vi "set IR test parameters.vi"(7 "IR Parameters":T1={"Voltage Level [V]"=1000, "Hi Limit [ohm]"=2500000.0, "Test Time [s] "=3.3, "Dwell Time [s]"=4.4, "Lo Limit [ohm]"=30000000000.0, "Ramp Time [s] "=1.1, "Fall Time [s]"=2.2} {"Voltage Level [V]" format="%.3p"; "Hi Limit [ohm]" format="%#_6p"; "Lo Limit [ohm]" format="%#_6p"}, 8 "error in (no error)":errorcluster, 10 "Step":T2 min=1 max=99 step=1, 11 "VISA Refnum in":refnum<visa-resource-name>) -> (0 "error out":errorcluster, 3 "VISA Refnum out":refnum<visa-resource-name>)   [LabVIEW 2025]
uses:
  Type Def/steps--ring.ctl
  Type Def/AC-DC-IR modes--ring.ctl
  Type Def/DC-IR modes--ring.ctl
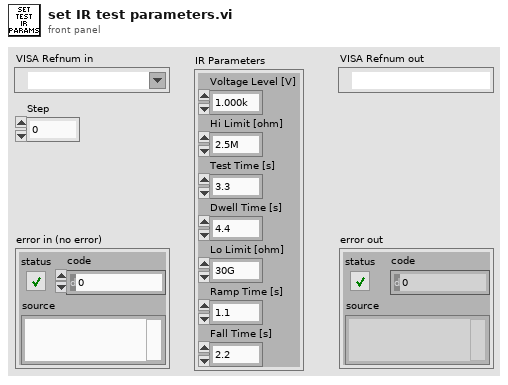
[diagram p1: front panel]
types:
  T1 = cluster{"Voltage Level [V]":u16, "Hi Limit [ohm]":dbl, "Test Time [s] ":dbl, "Dwell Time [s]":dbl, "Lo Limit [ohm]":dbl, "Ramp Time [s] ":dbl, "Fall Time [s]":dbl}
  T2 = typedef "steps--ring.ctl" = u8
  T3 = typedef "DC-IR modes--ring.ctl" = u16
  T4 = typedef "AC-DC-IR modes--ring.ctl" = u16
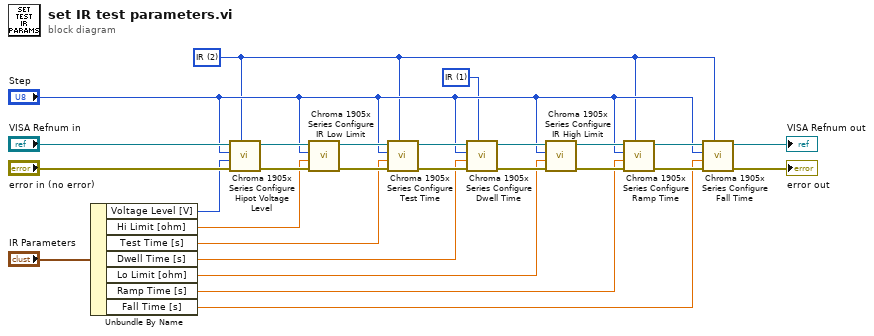
[diagram p0: block diagram]
diagram:
  w10 = T3 1 items=["DC", "IR"] ("Mode")
  w9 = T4 2 items=["AC", "DC", "IR"] ("Mode")
  n1 = Unbundle By Name("IR Parameters") -> ("Voltage Level [V]"=w7:u16, "Hi Limit [ohm]"=w6:dbl, "Test Time [s]"=w5:dbl, "Dwell Time [s]"=w4:dbl, "Lo Limit [ohm]"=w3:dbl, "Ramp Time [s]"=w2:dbl, "Fall Time [s]"=w1:dbl)
  n2 = call "Chroma 1905x Series Configure Hipot Voltage Level.vi"("Mode"=w9, "error in (no error)"="error in (no error)", "Voltage Level [V]"=w7, "Step"="Step", "VISA resource name"="VISA Refnum in") -> ("error out"=w18:errorcluster, "VISA resource name out"=w15:refnum<visa-resource-name>)  [unwired: 5 in]
  n3 = call "Chroma 1905x Series Configure IR Low Limit.vi"("error in (no error)"=w18, "Low Limit [ohm]"=w6, "Step"="Step", "VISA resource name"=w15) -> ("error out"=w21:errorcluster, "VISA resource name out"=w22:refnum<visa-resource-name>)  [unwired: 6 in]
  n4 = call "Chroma 1905x Series Configure Test Time.vi"("Mode"=w9, "error in (no error)"=w21, "Test Time [s]"=w5, "Step"="Step", "VISA resource name"=w22) -> ("error out"=w24:errorcluster, "VISA resource name out"=w12:refnum<visa-resource-name>)  [unwired: 5 in]
  n5 = call "Chroma 1905x Series Configure Dwell Time.vi"("Mode"=w10, "error in (no error)"=w24, "Dwell Time [s]"=w4, "Step"="Step", "VISA resource name"=w12) -> ("error out"=w23:errorcluster, "VISA resource name out"=w25:refnum<visa-resource-name>)  [unwired: 5 in]
  n6 = call "Chroma 1905x Series Configure IR High Limit.vi"("error in (no error)"=w23, "Hi Limit [ohm]"=w3, "Step"="Step", "VISA resource name"=w25) -> ("error out"=w27:errorcluster, "VISA resource name out"=w26:refnum<visa-resource-name>)  [unwired: 6 in]
  n7 = call "Chroma 1905x Series Configure Ramp Time.vi"("Mode"=w9, "error in (no error)"=w27, "Ramp Time [s]"=w2, "Step"="Step", "VISA resource name"=w26) -> ("error out"=w19:errorcluster, "VISA resource name out"=w20:refnum<visa-resource-name>)  [unwired: 5 in]
  n8 = call "Chroma 1905x Series Configure Fall Time.vi"("Mode"=w9, "error in (no error)"=w19, "Fall Time [s]"=w1, "Step"="Step", "VISA resource name"=w20) -> ("error out"=→"error out":errorcluster, "VISA resource name out"=→"VISA Refnum out":refnum<visa-resource-name>)  [unwired: 5 in]
